vi "data_processor.vi"(0 "data":waveform(dbl)[](array[waveform]), 1 "start time":timestamp, 5 "Active Analog Channel-Data Packages In":T2[](array[typedef]) {"Analog Input Channel"."Unit Conversion" format="%0.5f"; "Analog Input Channel"."TC Type" items=["J"=10072, "K"=10073, "N"=10077, "R"=10082, "S"=10085, "T"=10086, "B"=10047, "E"=10055]; "Analog Input Channel"."Sensor Offset" format="%0.5f"; "Analog Input Channel"."Sensor Max" format="%0.5f"; "Analog Input Channel"."Sensor Min" format="%0.5f"; "Analog Input Channel"."Maximum Value" format="%0.5f"; "Analog Input Channel"."Minimum Value" format="%0.5f"; "Analog Input Channel"."Terminal Configuration" items=["Default"=-1, "RSE"=10083, "NRSE"=10078, "Differential"=10106, "Pseudodifferential"=12529]}, 11 "error in":errorcluster) -> (4 "Analog Data Array":T1[](array[typedef]), 6 "Active Analog Channel-Data Packages Out":T2[](array[typedef]) {"Analog Input Channel"."Unit Conversion" format="%0.5f"; "Analog Input Channel"."TC Type" items=["J"=10072, "K"=10073, "N"=10077, "R"=10082, "S"=10085, "T"=10086, "B"=10047, "E"=10055]; "Analog Input Channel"."Sensor Offset" format="%0.5f"; "Analog Input Channel"."Sensor Max" format="%0.5f"; "Analog Input Channel"."Sensor Min" format="%0.5f"; "Analog Input Channel"."Maximum Value" format="%0.5f"; "Analog Input Channel"."Minimum Value" format="%0.5f"; "Analog Input Channel"."Terminal Configuration" items=["Default"=-1, "RSE"=10083, "NRSE"=10078, "Differential"=10106, "Pseudodifferential"=12529]}, 15 "error out":errorcluster)   [LabVIEW 2017]
uses:
  Box/Annular Flow/Jason/LabVIEW 2017/Input Channel Lists/analog_data_channel_pkg.ctl
  input_channel.ctl
  Box/Annular Flow/Jason/LabVIEW 2017/Input Channel Lists/analog_data.ctl
  <vilib>/Analysis/baseanly.llb/Mean (DBL).vi
  <vilib>/Waveform/WDTOps.llb/WDT Get Waveform Time Array DBL.vi
  <vilib>/gmath/NI_Gmath.lvlib
  <vilib>/Analysis/NI_AALBase.lvlib
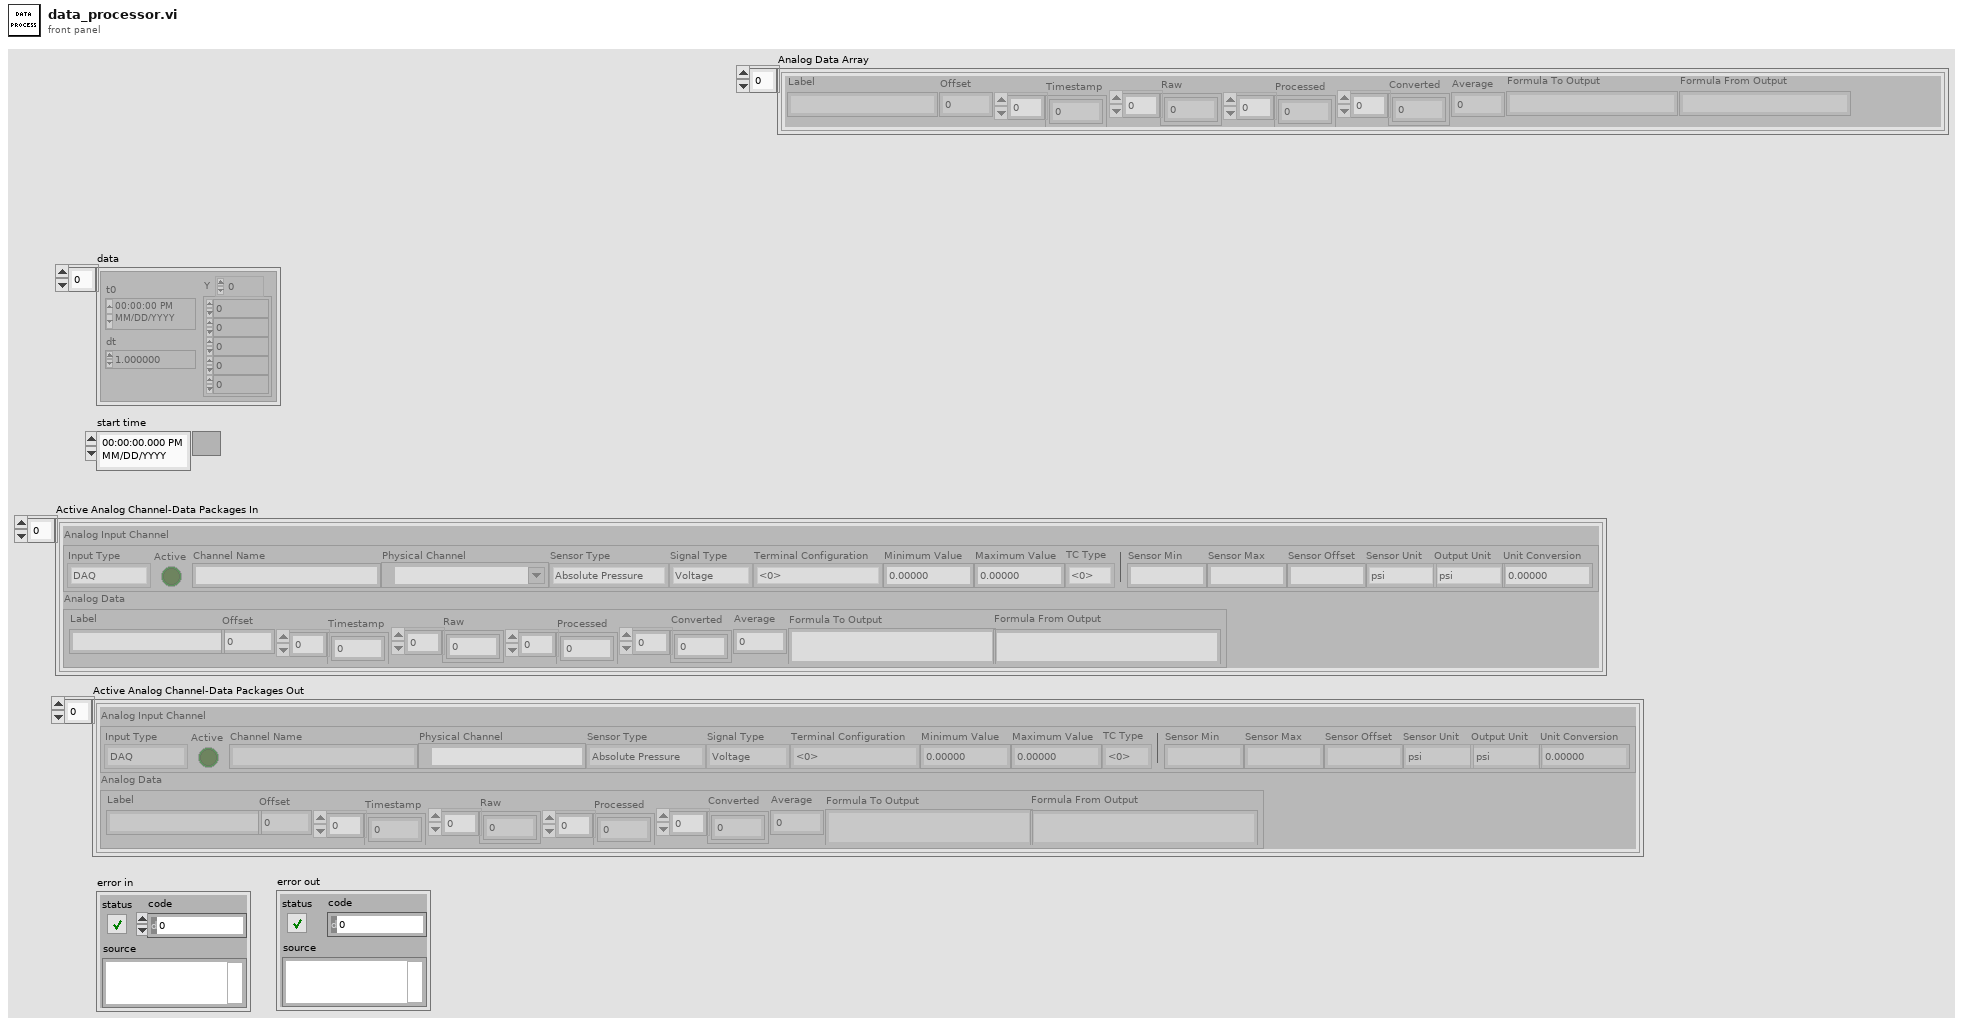
[diagram p1: front panel]
types:
  T1 = typedef "analog_data.ctl" = cluster{"Label":string, "Offset":dbl, "Timestamp":dbl[], "Raw":dbl[], "Processed":dbl[], "Converted":dbl[], "Average":dbl, "Formula To Output":string, "Formula From Output":string}
  T2 = typedef "analog_data_channel_pkg.ctl" = cluster{"Analog Input Channel":T3, "Analog Data":T1}
  T3 = typedef "input_channel.ctl" = cluster{"Channel Name":string, "Physical Channel":tag, "Sensor Type":enum16{"Absolute Pressure", "Gauge Pressure", "Differential Pressure", "Temperature", "Mass Flow Rate", "Density", "Other"}, "Signal Type":enum16{"Voltage", "Current", "Temperature"}, "Terminal Configuration":i32, "Minimum Value":dbl, "Maximum Value":dbl, "TC Type":i32, "Sensor Min":dbl, "Sensor Max":dbl, "Sensor Offset":dbl, "Sensor Unit":enum16{"psi", "Pa", "inH2O", "inHg", "C", "K", "g/s", "g/cm3", "Volt", "Amp", ""}, "Output Unit":enum16{"psi", "Pa", "inH2O", "inHg", "C", "K", "g/s", "g/cm3", "Volt", "Amp", ""}, "Unit Conversion":dbl, "Active":bool, "Input Type":enum16{"DAQ", "Add-On"}}
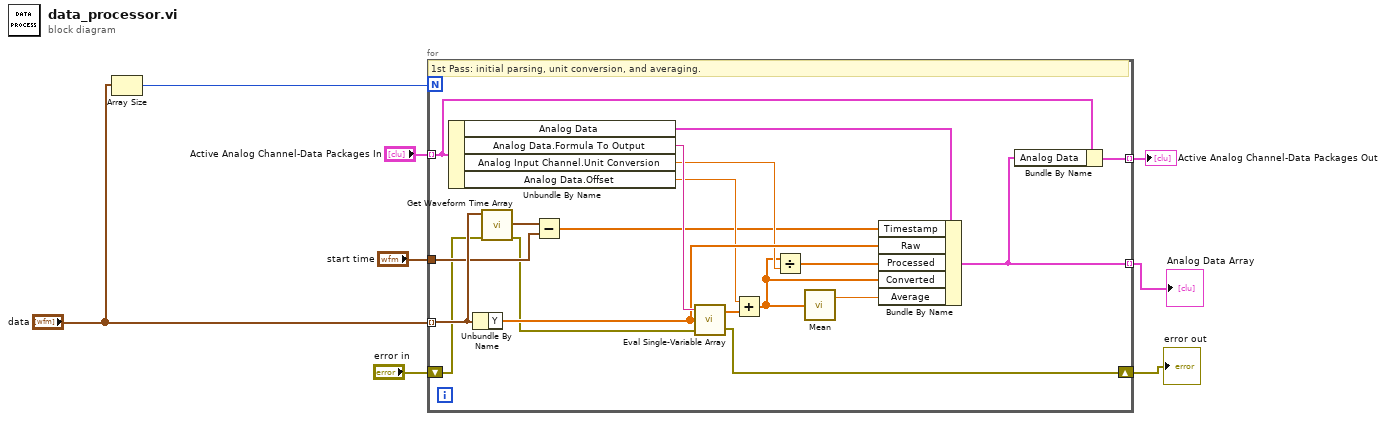
[diagram p0: block diagram]
diagram:
  n1 = Array Size(array="data") -> (size(s)=w2:i32)
  n2 = for {
    N: w2 -> [_]
    tunnel: "Active Analog Channel-Data Packages In" -> [w14] mode=indexing
    tunnel: "data" -> [w26] mode=indexing
    tunnel: [w13] -> w5 mode=indexing
    tunnel: "start time" -> [w16]
    tunnel: [w12] -> w6 mode=indexing
    shift-right: [w9] -> w1
    shift-left: "error in" -> [w11]
    # "1st Pass: initial parsing, unit conversion, and averaging."
    n3 = Unbundle By Name(w14) -> ("Analog Data"=w27:T1, "Analog Data.Formula To Output"=w25:string, "Analog Input Channel.Unit Conversion"=w22:dbl, "Analog Data.Offset"=w18:dbl)
    n4 = Unbundle By Name(w26) -> ("Y"=w24:dbl[])
    n5 = call-poly <vilib>:"Get Waveform Time Array.vi"("error in (no error)"=w11, "waveform in"=w26) -> ("error out"=w10:errorcluster, "X array"=w17:timestamp[])  [unwired: 8 in]
    n6 = Subtract(x=w17, y=w16) -> (x-y=w15:dbl[])
    n7 = call <vilib>:"Eval Single-Variable Array.vi"("error in (no error)"=w10, "X Values"=w24, "formula"=w25) -> ("error out"=w9:errorcluster, "Y Values"=w20:dbl[])
    n8 = Add(x=w18, y=w20) -> (x+y=w19:dbl[])
    n9 = Divide(x=w19, y=w22) -> (x/y=w21:dbl[])
    n10 = call-poly <vilib>:"Mean.vi"("X"=w19) -> ("mean"=w23:dbl)  [unwired: 1 out]
    n11 = Bundle By Name(cluster=w27, "Timestamp"=w15, "Raw"=w24, "Processed"=w21, "Converted"=w19, "Average"=w23) -> (w13:T1)
    n12 = Bundle By Name(cluster=w14, "Analog Data"=w13) -> (w12:T2)
  }
  "Active Analog Channel-Data Packages Out" <- w6
  "error out" <- w1
  "Analog Data Array" <- w5
